vi "Save Recording FGV.vi"(6 "Command":T1, 8 "Save":bool) -> (0 "Save?":bool)   [LabVIEW 2015]
uses:
  TypeDefs Host/Open Audio FGV Enum.ctl
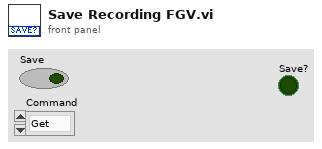
[diagram p1: front panel]
types:
  T1 = typedef "Open Audio FGV Enum.ctl" = enum16{"Get", "Set"}
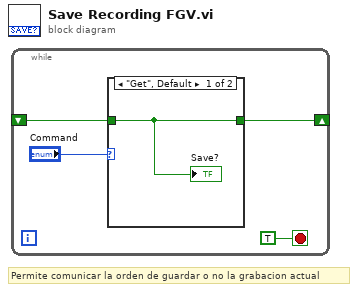
[diagram p0: block diagram]
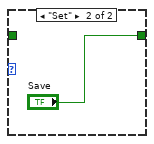
[diagram p2: hidden frame]
diagram:
  # "Permite comunicar la orden de guardar o no la grabacion actual"
  n1 = while {
    shift-right: [w2] -> _
    shift-left: _ -> [w1]
    stop <- TRUE stop-if-true
    n2 = case shown="\"Get\", Default" "Command" {
      tunnel: [w5 "Save"] -> w2
      tunnel: w1 -> [w5 _]
      frame "Get", Default {
        "Save?" <- w5
      }
      frame "Set" {
      }
    }
  }
